vi "ExFilterWheel2.vi"() -> ()   [LabVIEW 2010]
panel:
  in  "Select Filter Wheel":i16=1 min=1 max=4 step=1
  out "Number of Filter Wheels":i16
  in  "?":bool
  out "Filter Wheel Open":bool
  out "Number Of Filters":i16=1 min=1 step=1
  in  "?":bool
  in  "?":bool
  out "Filter":i16=1 min=1 step=1
  in  "?":bool
  in  "?":bool
  in  "?":bool
  in  "Filter":i16=1 min=1 max=100 step=1
  out "error out":errorcluster
  in  "error in":errorcluster
  # "ExFilterWheel2.vi\n(Filter wheel control through spectrometer)\nThis example shows how access a filter wheel via the spectrometer handle.\nNot all commands may be available for all filter wheels."
  # "The number of filters is set in the .ini file"
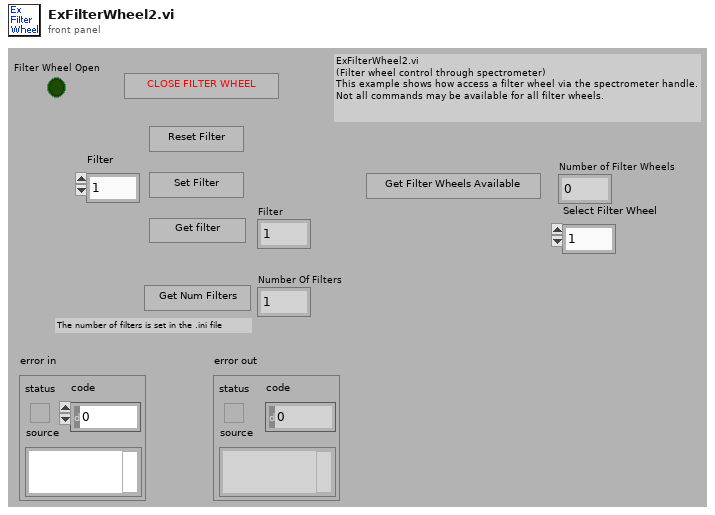
[diagram p1: front panel]
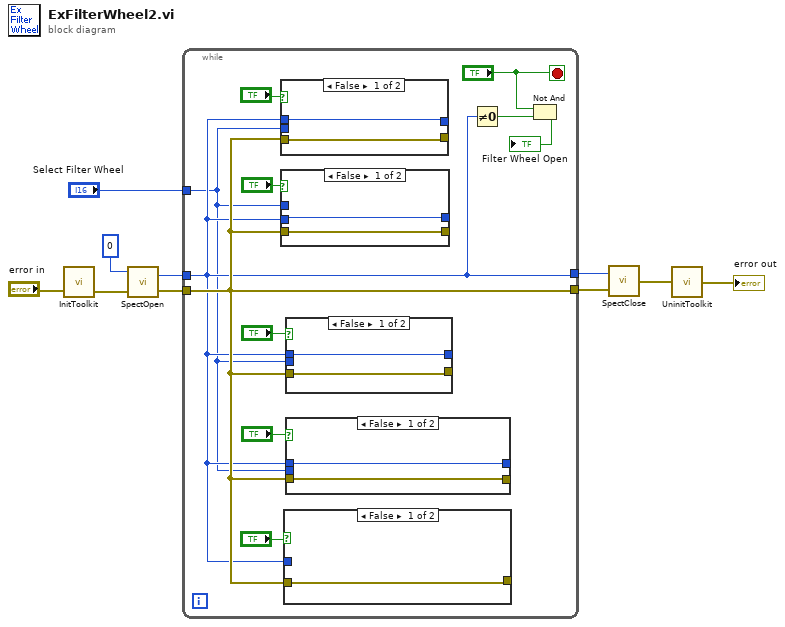
[diagram p0: block diagram]
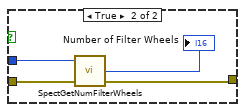
[diagram p2: hidden frame]
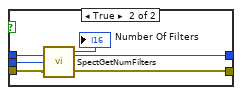
[diagram p3: hidden frame]
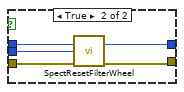
[diagram p4: hidden frame]
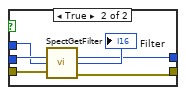
[diagram p5: hidden frame]
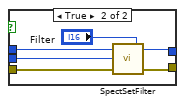
[diagram p6: hidden frame]
diagram:
  n1 = call <userlib>:"InitToolkit.vi"("error in"="error in") -> ("error out"=w9:errorcluster)
  n2 = call <userlib>:"SpectOpen.vi"("error in"=w9, "Spectrometer ID"=0) -> ("error out"=w5:errorcluster, "Spectrometer Handle"=w2:u32)  [unwired: 1 in]
  n3 = while {
    tunnel: w2 -> [w12]
    tunnel: w5 -> [w13]
    tunnel: [w12] -> w4
    tunnel: [w13] -> w3
    tunnel: "Select Filter Wheel" -> [w11]
    stop <- "?" stop-if-true
    n4 = case shown="False" "?" {
      tunnel: [w50 w57] -> _
      tunnel: [w51 w56] -> _
      tunnel: w12 -> [w51 w55]
      tunnel: w13 -> [w50 w54]
      tunnel: w11 -> [_ w53]
      frame False {
      }
      frame True {
        n5 = call <userlib>:"SpectSetFilter.vi"("Filter Number"="Filter", "error in"=w54, "Filter Wheel Number"=w53, "Spectrometer Handle"=w55) -> ("error out"=w57:errorcluster, "Spectrometer Handle"=w56:u32)
      }
    }
    n6 = case shown="False" "?" {
      tunnel: w12 -> [w43 w49]
      tunnel: w13 -> [w42 w48]
      tunnel: [w42 w47] -> _
      tunnel: [w43 w45] -> _
      tunnel: w11 -> [_ w44]
      frame False {
      }
      frame True {
        n7 = call <userlib>:"SpectGetFilter.vi"("error in"=w48, "Filter Wheel Number"=w44, "Spectrometer Handle"=w49) -> ("error out"=w47:errorcluster, "Filter Number"=→"Filter":i16, "Spectrometer Handle"=w45:u32)
      }
    }
    n8 = case shown="False" "?" {
      tunnel: w13 -> [w22 w26]
      tunnel: [w22 w25] -> _
      tunnel: w12 -> [_ w24]
      frame False {
      }
      frame True {
        n9 = call <userlib>:"SpectGetNumFilterWheels.vi"("error in"=w26, "Spectrometer Handle"=w24) -> ("error out"=w25:errorcluster, "Filter Number"=→"Number of Filter Wheels":i16)  [unwired: 1 in, 1 out]
      }
    }
    n10 = case shown="False" "?" {
      tunnel: w13 -> [w35 w39]
      tunnel: w12 -> [w36 w41]
      tunnel: [w36 w40] -> _
      tunnel: [w35 w38] -> _
      tunnel: w11 -> [_ w37]
      frame False {
      }
      frame True {
        n11 = call <userlib>:"SpectResetFilterWheel.vi"("error in"=w39, "Filter Wheel"=w37, "Spectrometer Handle"=w41) -> ("error out"=w38:errorcluster, "Spectrometer Handle"=w40:u32)  [unwired: 1 in]
      }
    }
    n12 = case shown="False" "?" {
      tunnel: w12 -> [w28 w33]
      tunnel: [w28 w32] -> _
      tunnel: w13 -> [w27 w31]
      tunnel: [w27 w30] -> _
      tunnel: w11 -> [_ w29]
      frame False {
      }
      frame True {
        n13 = call <userlib>:"SpectGetNumFilters.vi"("error in"=w31, "Filter Wheel"=w29, "Spectrometer Handle"=w33) -> ("error out"=w30:errorcluster, "Number of Filters"=→"Number Of Filters":i16, "Spectrometer Handle"=w32:u32)
      }
    }
    n14 = Not Equal To 0?(x=w12) -> (x != 0?=w17:bool)
    n15 = Not And(1:w17, 2:"?") -> (0:→"Filter Wheel Open":bool)
  }
  n16 = call <userlib>:"SpectClose.vi"("error in"=w3, "Spectrometer Handle"=w4) -> ("error out"=w6:errorcluster)
  n17 = call <userlib>:"UninitToolkit.vi"("error in"=w6) -> ("error out"=→"error out":errorcluster)
